vi "BUILD_post build add to repo.vi"() -> ()   [LabVIEW 2013]
panel:
  out "error out":errorcluster
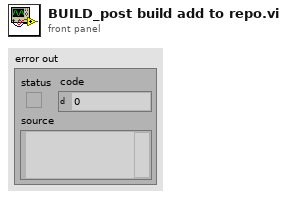
[diagram p1: front panel]
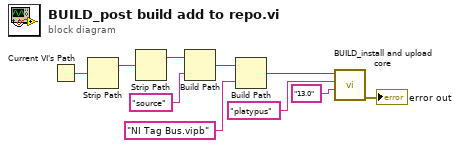
[diagram p0: block diagram]
diagram:
  n1 = Current VI's Path() -> (path=w10:path)
  n2 = Strip Path(path=w10) -> (stripped path=w9:path)  [unwired: 1 out]
  n3 = Strip Path(path=w9) -> (stripped path=w7:path)  [unwired: 1 out]
  n4 = Build Path(base path=w7, name or relative path="source") -> (appended path=w2:path)
  n5 = Build Path(base path=w2, name or relative path="NI Tag Bus.vipb") -> (appended path=w1:path)
  n6 = call "BUILD_install and upload core.vi"("LabVIEW Version"="13.0", "Repository Name"="platypus", "appended path"=w1) -> ("error out"=→"error out":errorcluster)  [unwired: 8 in]
